vi "K2450 Ramp Voltage.vi"() -> ()   [LabVIEW 2020]
panel:
  in  "Clone":bool
  out "Time Remaining":dbl=60.0 format="%<%H:%M:%S>t"
  out "Output Voltage":dbl format="%_4g"
  in  "Time (Hr:Min:Sec)":dbl=60.0 step=1.0 format="%<%H:%M:%S>t"
  in  "Stop Voltage":dbl format="%.6g"
  in  "Start Ramp":bool
  in  "Update Time":dbl=0.1 format="%.3g"
  in  "stop":bool
  in  "VISA resource name":refnum<visa-resource-name>
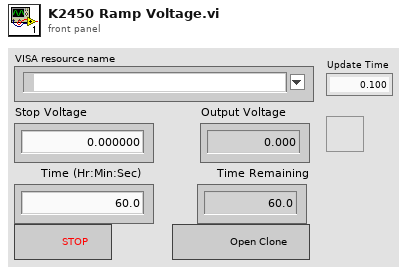
[diagram p1: front panel]
types:
  T1 = enum8{"Enabled", "Disabled", "Disabled and Grayed Out"}
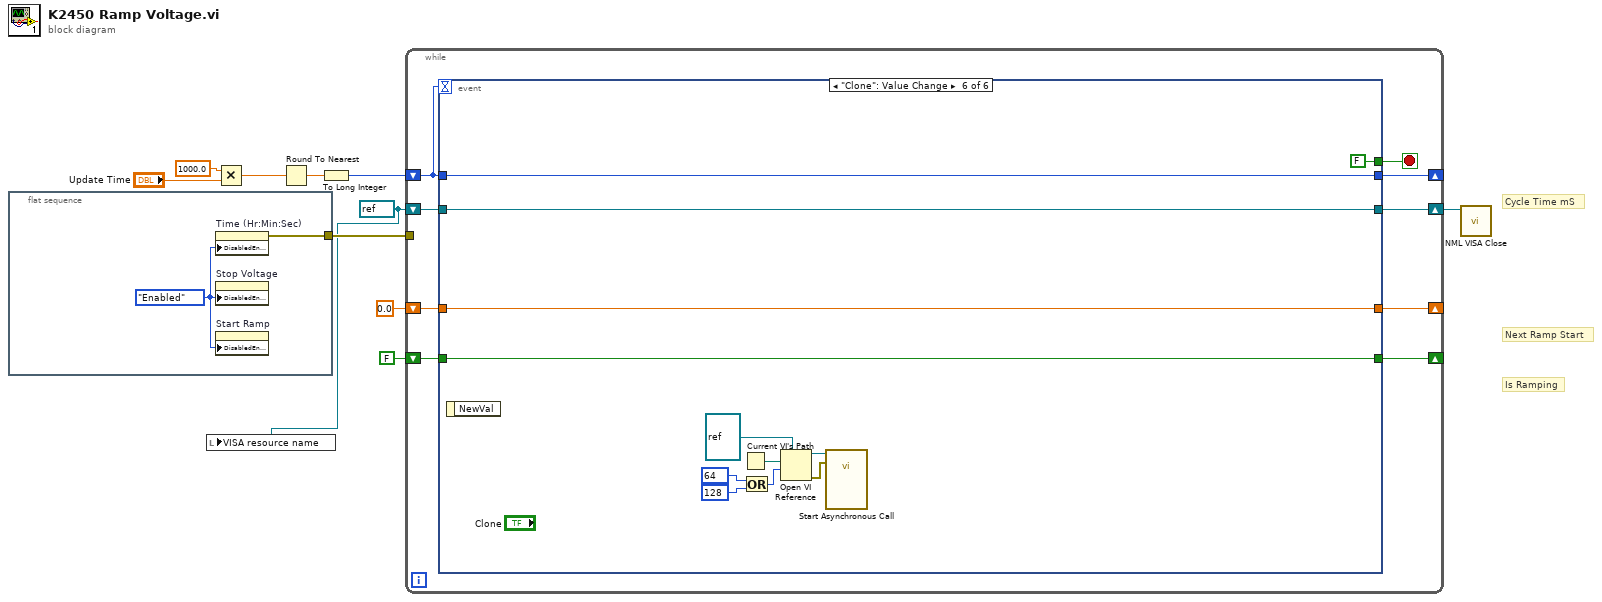
[diagram p0: block diagram]
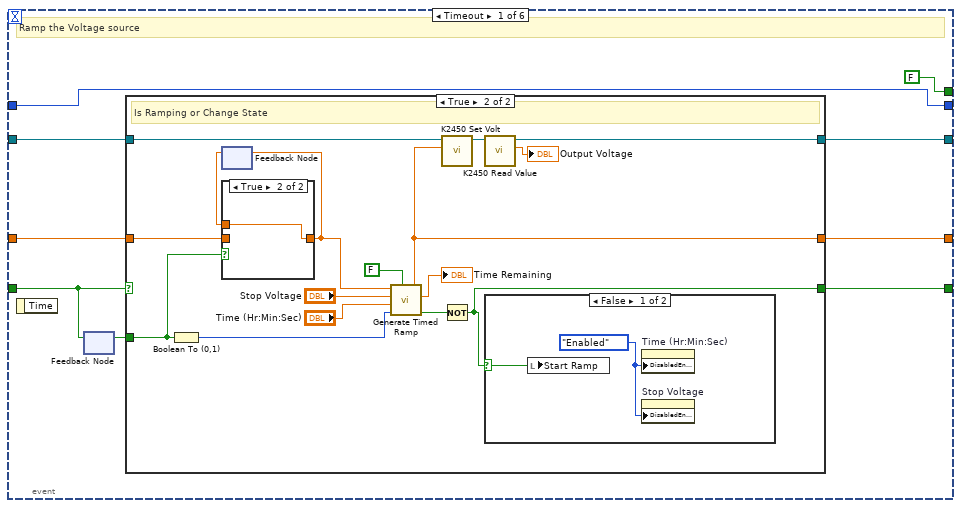
[diagram p2: hidden frame]
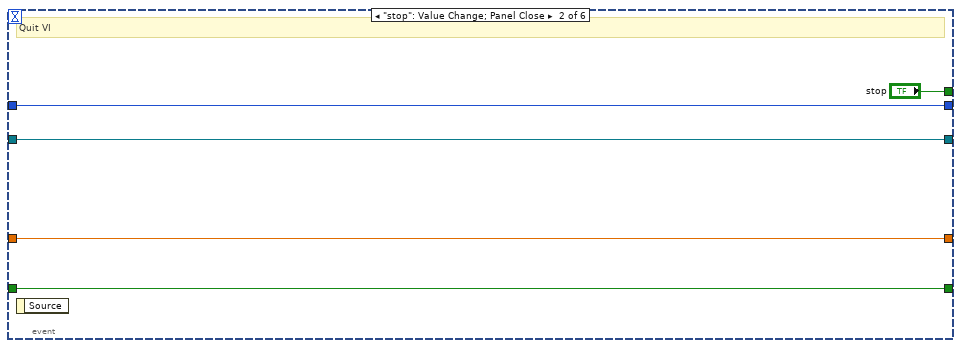
[diagram p6: hidden frame]
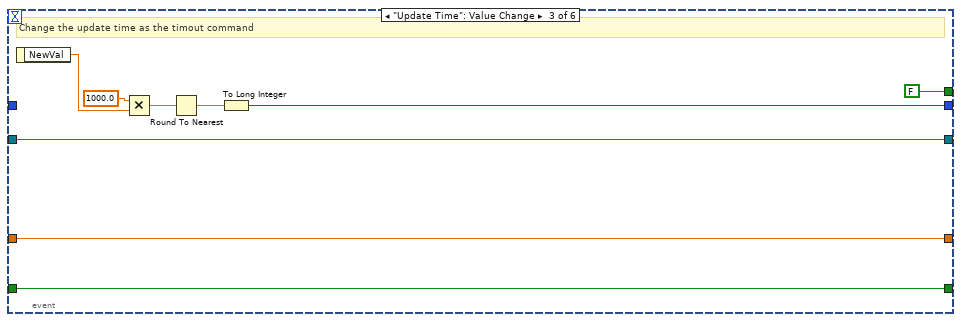
[diagram p7: hidden frame]
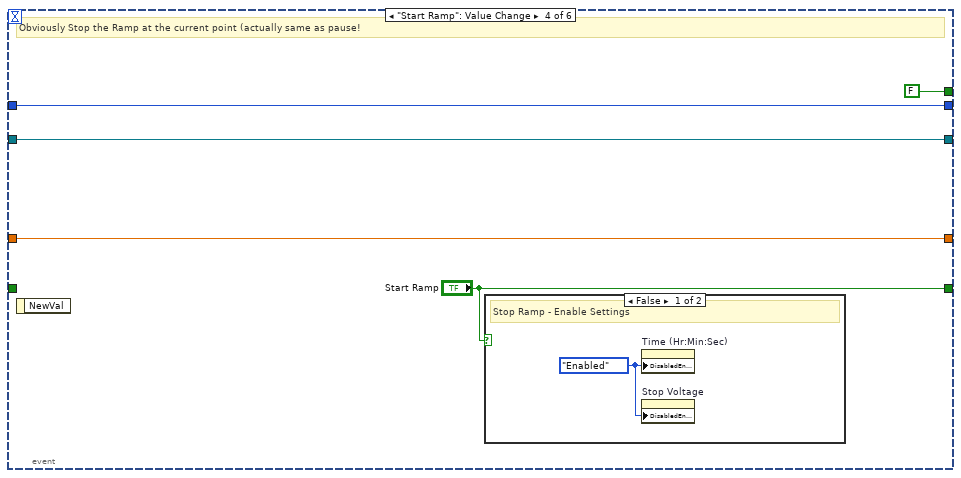
[diagram p8: hidden frame]
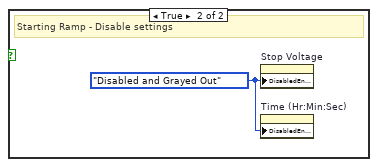
[diagram p9: hidden frame]
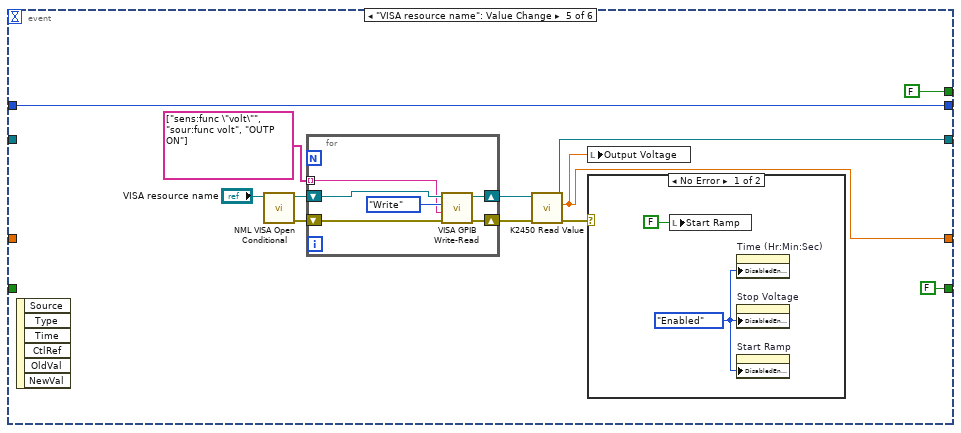
[diagram p10: hidden frame]
diagram:
  w1 = refnum<visa-resource-name> refnum ("dup VISA Session")
  # "Is Ramping"
  # "Next Ramp Start"
  # "Cycle Time mS"
  n1 = flat-sequence {
    tunnel: [w11] -> w2
    frame #0 {
      w12 = T1."Enabled" ("Disabled")
      n2 = property on="Time (Hr:Min:Sec)" class="DigNum (strict)"("DisabledEnum"=w12) -> (error out=w11:errorcluster)  [unwired: 2 in, 1 out]
      n3 = property on="Stop Voltage" class="DigNum (strict)"("DisabledEnum"=w12) -> ()  [unwired: 2 in, 2 out]
      n4 = property on="Start Ramp" class="Bool (strict)"("DisabledEnum"=w12) -> ()  [unwired: 2 in, 2 out]
    }
  }
  n5 = local write "VISA resource name"(w1) -> ()
  n6 = Multiply(x=1000.0, y="Update Time") -> (x*y=w9:dbl)
  n7 = Round To Nearest(number=w9) -> (nearest integer value=w7:dbl)
  n8 = To Long Integer(number=w7) -> (32bit integer=w6:i32)
  n9 = while {
    shift-right: [w17] -> w5
    shift-left: w1 -> [w18]
    shift-right: [w14] -> _
    shift-left: 0.0 ("Voitage 2450") -> [w13]
    shift-right: [w19] -> _
    shift-left: w6 -> [w20]
    shift-right: [w15] -> _
    shift-left: FALSE -> [w16]
    tunnel: w2 -> [_]
    stop <- w21 stop-if-true
    n10 = event shown="[5] \"Clone\": Value Change" {
      selector: _ -> [_ _ _ _ _ _]
      dyn-events: _ -> [_ _ _ _ _ _]
      timeout: w20 -> [_ _ _ _ _ _]
      tunnel: [FALSE ("stop") "stop" FALSE ("stop") FALSE ("stop") FALSE ("stop") FALSE ("stop")] -> w21
      tunnel: w20 -> [w30 w57 _ w71 w79 w105]
      tunnel: [w30 w57 w63 w71 w79 w105] -> w19
      tunnel: w18 -> [w29 w54 w60 w70 _ w106]
      tunnel: [w28 w54 w60 w70 w80 w106] -> w17
      tunnel: w16 -> [w23 w56 w61 _ _ w102]
      tunnel: [w26 w56 w61 "Start Ramp" FALSE ("Start Ramp") w102] -> w15
      tunnel: [w24 w55 w59 w69 w76 w103] -> w14
      tunnel: w13 -> [w25 w55 w59 w69 _ w103]
      event Timeout {
        # "Ramp the Voltage source"
        n11 = event-data() -> ()  [unwired: 1 in, 1 out]
        n12 = feedback-in #1(w23) -> ()
        n13 = feedback #1() -> (w22:bool)  [unwired: 1 in]
        n14 = case shown="True" w23 {
          selector: w23 -> [w31 _]
          tunnel: w29 -> [w33 w48]
          tunnel: [w33 w41] -> w28
          tunnel: [w31 w39] -> w26
          tunnel: w25 -> [w32 w37]
          tunnel: [w32 w43] -> w24
          tunnel: w22 -> [_ w38]
          frame False {
            # "Idle"
          }
          frame True {
            # "Is Ramping or Change State"
            n15 = Boolean To (0,1)(Boolean=w38) -> (0, 1=w47:i16)
            n16 = feedback #2() -> (w35:dbl)  [unwired: 1 in]
            n17 = case shown="True" w38 {
              tunnel: w37 -> [w50 _]
              tunnel: [w50 w51] -> w36
              tunnel: w35 -> [_ w51]
              frame False {
              }
              frame True {
              }
            }
            n18 = feedback-in #2(w36) -> ()
            n19 = call "Generate Timed Ramp.vi"("Log"=FALSE, "Point #"=w47, "Time (Hr:Min:Sec)"="Time (Hr:Min:Sec)", "Stop"="Stop Voltage", "Start"=w36) -> ("Stop"=w46:bool, "Time Remaining"=→"Time Remaining":dbl, "Output"=w43:dbl)  [unwired: 1 out]
            n20 = call "K2450 Set Volt.vi"("Voltage 2450"=w43, "VISA resource name"=w48) -> ("dup VISA Session"=w42:refnum<visa-resource-name>)  [unwired: 8 in, 1 out]
            n21 = Not(x=w46) -> (.not. x?=w39:bool)
            n22 = call "K2450 Read Value.vi"("VISA resource name"=w42) -> ("Value 2450"=→"Output Voltage":dbl, "dup VISA Session"=w41:refnum<visa-resource-name>)  [unwired: 8 in, 1 out]
            n23 = case shown="False" w39 {
              selector: w39 -> [w53 _]
              frame False {
                w52 = T1."Enabled" ("Disabled")
                n24 = local write "Start Ramp"(w53) -> ()
                n25 = property on="Time (Hr:Min:Sec)" class="DigNum (strict)"("DisabledEnum"=w52) -> ()  [unwired: 2 in, 2 out]
                n26 = property on="Stop Voltage" class="DigNum (strict)"("DisabledEnum"=w52) -> ()  [unwired: 2 in, 2 out]
              }
              frame True {
              }
            }
          }
        }
      }
      event "stop": Value Change; Panel Close {
        # "Quit VI"
        n27 = event-data() -> ()  [unwired: 1 in, 1 out]
      }
      event "Update Time": Value Change {
        # "Change the update time as the timout command"
        n28 = event-data() -> ("NewVal"=w64:dbl)  [unwired: 1 in]
        n29 = Multiply(x=1000.0, y=w64) -> (x*y=w65:dbl)
        n30 = Round To Nearest(number=w65) -> (nearest integer value=w67:dbl)
        n31 = To Long Integer(number=w67) -> (32bit integer=w63:i32)
      }
      event "Start Ramp": Value Change {
        # "Obviously Stop the Ramp at the current point (actually same as pause!"
        n32 = event-data() -> ()  [unwired: 1 in, 1 out]
        n33 = case shown="False" "Start Ramp" {
          frame False {
            w73 = T1."Enabled" ("Disabled")
            # "Stop Ramp - Enable Settings"
            n34 = property on="Time (Hr:Min:Sec)" class="DigNum (strict)"("DisabledEnum"=w73) -> ()  [unwired: 2 in, 2 out]
            n35 = property on="Stop Voltage" class="DigNum (strict)"("DisabledEnum"=w73) -> ()  [unwired: 2 in, 2 out]
          }
          frame True {
            w74 = T1."Disabled and Grayed Out" ("Disabled")
            # "Starting Ramp - Disable settings"
            n36 = property on="Stop Voltage" class="DigNum (strict)"("DisabledEnum"=w74) -> ()  [unwired: 2 in, 2 out]
            n37 = property on="Time (Hr:Min:Sec)" class="DigNum (strict)"("DisabledEnum"=w74) -> ()  [unwired: 2 in, 2 out]
          }
        }
      }
      event "VISA resource name": Value Change {
        n38 = event-data() -> ()  [unwired: 1 in, 6 out]
        n39 = call "NML VISA Open Conditional.vi"("VISA resource name"="VISA resource name") -> ("error out"=w86:errorcluster, "dup VISA Session"=w83:refnum<visa-resource-name>)  [unwired: 8 in, 1 out]
        n40 = for {
          shift-right: [w92] -> w84
          shift-left: w83 -> [w90]
          shift-right: [w93] -> w85
          shift-left: w86 -> [w91]
          tunnel: string[] ["sens:func \"volt\"", "sour:func volt", "OUTP ON"] -> [w89] mode=indexing
          n41 = call "VISA GPIB Write-Read.vi"("error in (no error)"=w91, "Command"=w89, "Action"=enum16{"Write", "Read", "Write & Read"}."Write", "VISA resource name"=w90) -> ("error out"=w93:errorcluster, "dup VISA Session"=w92:refnum<visa-resource-name>)  [unwired: 4 in, 2 out]
        }
        n42 = call "K2450 Read Value.vi"("error in (no error)"=w85, "VISA resource name"=w84) -> ("error out"=w77:errorcluster, "Value 2450"=w76:dbl, "dup VISA Session"=w80:refnum<visa-resource-name>)  [unwired: 7 in]
        n43 = local write "Output Voltage"(w76) -> ()
        n44 = case shown="No Error" w77 {
          frame No Error {
            w88 = T1."Enabled" ("Disabled")
            n45 = local write "Start Ramp"(FALSE ("Start Ramp")) -> ()
            n46 = property on="Time (Hr:Min:Sec)" class="DigNum (strict)"("DisabledEnum"=w88) -> ()  [unwired: 2 in, 2 out]
            n47 = property on="Stop Voltage" class="DigNum (strict)"("DisabledEnum"=w88) -> ()  [unwired: 2 in, 2 out]
            n48 = property on="Start Ramp" class="Bool (strict)"("DisabledEnum"=w88) -> ()  [unwired: 2 in, 2 out]
          }
          frame Error {
          }
        }
      }
      event "Clone": Value Change {
        n49 = event-data() -> ()  [unwired: 1 in, 1 out]
        n50 = Current VI's Path() -> (path=w98:path)
        n51 = Or(x=64, y=128) -> (x .or. y?=w95:i32)
        n52 = Open VI Reference(type specifier VI Refnum (for type only)=refnum<vi> refnum, vi path=w98, options=w95) -> (vi reference=w101:refnum<vi>, error out=w100:errorcluster)  [unwired: 3 in]
        n53 = call-by-ref "Start Asynchronous Call"(reference=w101, error in=w100) -> ()  [unwired: 12 in, 2 out]
      }
    }
  }
  n54 = call "NML VISA Close.vi"("VISA resource name"=w5) -> ()  [unwired: 10 in, 1 out]
